vi "Post-Build Custom Action.vi"(10 "Variant":variant) -> (0 "error out":errorcluster)   [LabVIEW 2019]
uses:
  lvsrc/PostBuildSupport/PostBuildSupport.lvclass
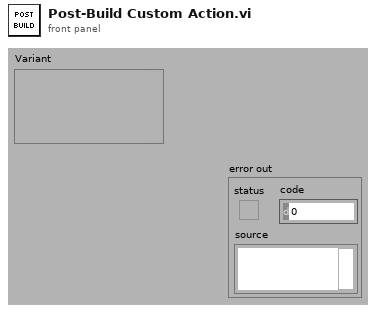
[diagram p1: front panel]
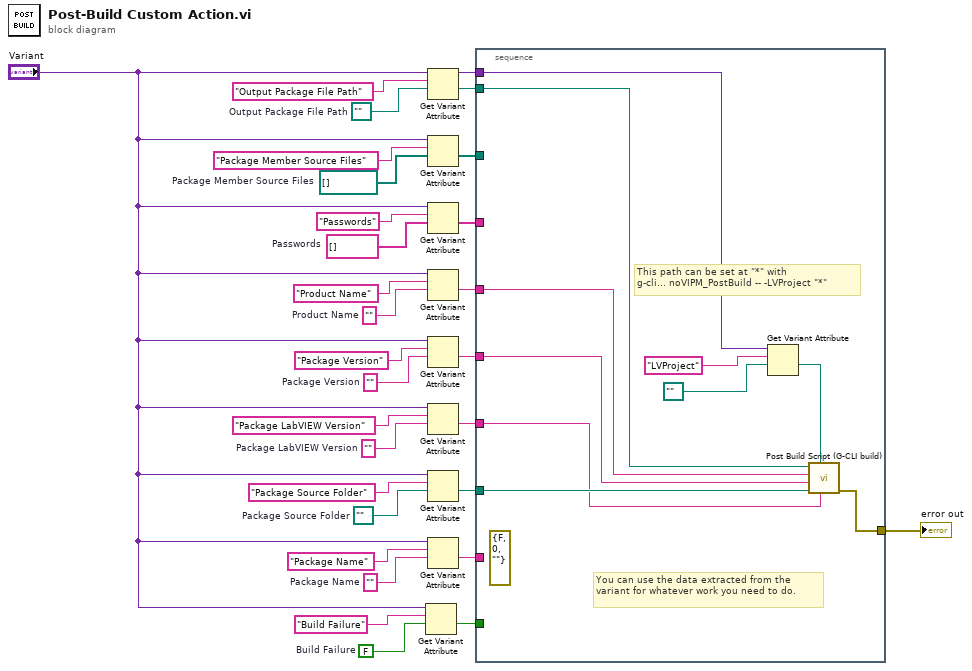
[diagram p0: block diagram]
diagram:
  w5 = FALSE  # Build Failure
  w15 = path ""  # Package Source Folder
  w16 = ""  # Package Name
  w19 = ""  # Package LabVIEW Version
  w21 = ""  # Package Version
  w23 = ""  # Product Name
  w25 = string[] []  # Passwords
  w27 = path[] []  # Package Member Source Files
  w29 = path ""  # Output Package File Path
  n1 = Get Variant Attribute(Variant="Variant", name="Build Failure", default value (empty Variant)=w5) -> (value=w3:bool)  [unwired: 1 in, 3 out]
  n2 = Get Variant Attribute(Variant="Variant", name="Output Package File Path", default value (empty Variant)=w29) -> (duplicate Variant=w1:variant, value=w14:path)  [unwired: 1 in, 2 out]
  n3 = Get Variant Attribute(Variant="Variant", name="Package Member Source Files", default value (empty Variant)=w27) -> (value=w13:path[])  [unwired: 1 in, 3 out]
  n4 = Get Variant Attribute(Variant="Variant", name="Passwords", default value (empty Variant)=w25) -> (value=w12:string[])  [unwired: 1 in, 3 out]
  n5 = Get Variant Attribute(Variant="Variant", name="Product Name", default value (empty Variant)=w23) -> (value=w11:string)  [unwired: 1 in, 3 out]
  n6 = Get Variant Attribute(Variant="Variant", name="Package Version", default value (empty Variant)=w21) -> (value=w10:string)  [unwired: 1 in, 3 out]
  n7 = Get Variant Attribute(Variant="Variant", name="Package LabVIEW Version", default value (empty Variant)=w19) -> (value=w9:string)  [unwired: 1 in, 3 out]
  n8 = Get Variant Attribute(Variant="Variant", name="Package Source Folder", default value (empty Variant)=w15) -> (value=w8:path)  [unwired: 1 in, 3 out]
  n9 = Get Variant Attribute(Variant="Variant", name="Package Name", default value (empty Variant)=w16) -> (value=w7:string)  [unwired: 1 in, 3 out]
  n10 = stacked-sequence {
    tunnel: w14 -> [w40]
    tunnel: w13 -> [_]
    tunnel: w12 -> [_]
    tunnel: w11 -> [w39]
    tunnel: w10 -> [w38]
    tunnel: w9 -> [w35]
    tunnel: w8 -> [w37]
    tunnel: w7 -> [_]
    tunnel: w3 -> [_]
    tunnel: [w36] -> w2
    tunnel: w1 -> [w32]
    frame #0 {
      (unwired) errorcluster {"status"=FALSE, "code"=0, "source"=""} ("error in")
      # "This path can be set at \"*\" with\ng-cli... noVIPM_PostBuild -- -LVProject \"*\""
      # "You can use the data extracted from the variant for whatever work you need to do."
      n11 = Get Variant Attribute(Variant=w32, name="LVProject", default value (empty Variant)=path "" ("Project File Path")) -> (value=w31:path)  [unwired: 1 in, 3 out]
      n12 = call "Post Build Script (G-CLI build).vi"("Package LabVIEW Version (19.0 (32-bit))"=w35, "Project File Path"=w31, "Package Source Folder"=w37, "Package Version (major.minor.patch.build)"=w38, "Product Name"=w39, "Output Package File Path"=w40) -> ("error out"=w36:errorcluster)  [unwired: 5 in]
    }
  }
  "error out" <- w2
